vi "MH-Enqueue Message.vi"(0 "MH Queue in":refnum<queue>, 5 "Message":string, 9 "Data":variant, 11 "error in (no error)":errorcluster) -> (4 "MH Queue out":refnum<queue>, 15 "error out":errorcluster)   [LabVIEW 2020]
uses:
  MH-Message.ctl
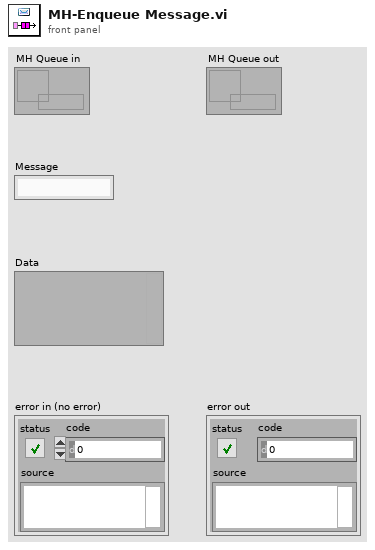
[diagram p1: front panel]
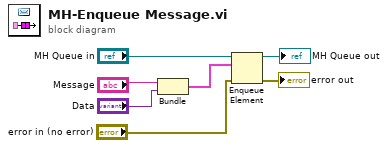
[diagram p0: block diagram]
diagram:
  n1 = Bundle("Message"="Message", "Data"="Data") -> (w4:cluster{"Message":string, "Data":variant})  [unwired: 1 in]
  n2 = Enqueue Element(queue="MH Queue in", element=w4, error in (no error)="error in (no error)") -> (queue out=→"MH Queue out":refnum<queue>, error out=→"error out":errorcluster)  [unwired: 1 in, 1 out]
